vi "Read Meta Data.vi"(11 "Tree Data In":refnum<class "Tree Data.lvclass">) -> (1 "Meta Data":string, 3 "Tree Data Out":refnum<class "Tree Data.lvclass">)   [LabVIEW 2020, in "NI_VIAnCFGDataStructure.lvlib" / "Tree Data.lvclass"]
doc: "Write the Meta Data associated with this Tree Data type. This can store any information."
uses:
  <vilib>/addons/analyzer/VIAnCFGDataStructure/Tree Data/Tree Data.lvclass
  <vilib>/addons/analyzer/VIAnCFGDataStructure/Tree Data/Tree Data.lvclass/Tree Data.ctl
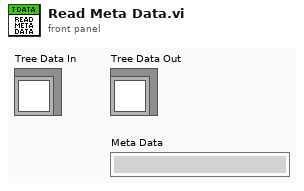
[diagram p1: front panel]
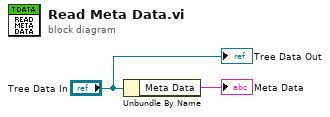
[diagram p0: block diagram]
diagram:
  n1 = Unbundle By Name("Tree Data In") -> ("Meta Data"=→"Meta Data":string)
  "Tree Data Out" <- "Tree Data In"
